vi "Valves2Linx.vi"(8 "error in (no error)":errorcluster, 11 "Valve (A1-C8),\n comma separated":string) -> (0 "error out":errorcluster, 2 "Array":bool[](array[boolean]), 3 "Array 2":i32[](array[numeric]))   [LabVIEW 2018]
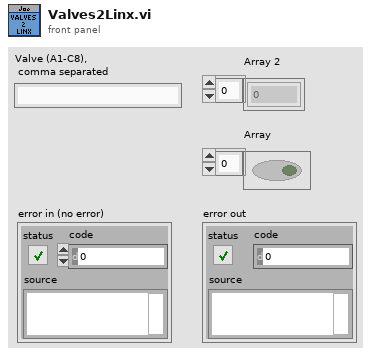
[diagram p1: front panel]
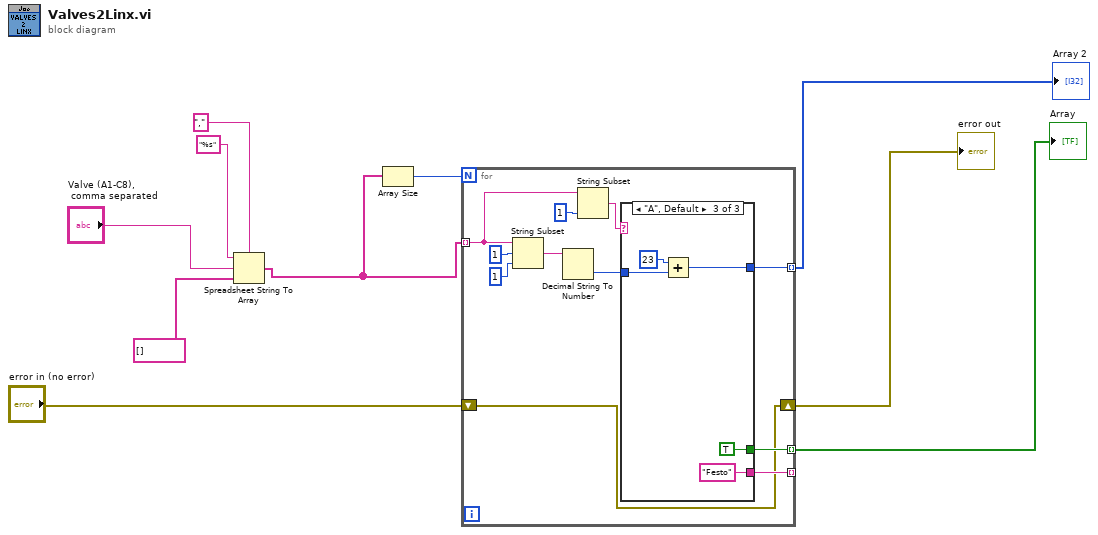
[diagram p0: block diagram]
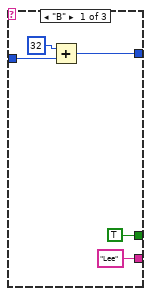
[diagram p2: hidden frame]
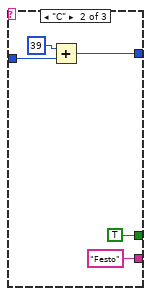
[diagram p3: hidden frame]
diagram:
  n1 = Spreadsheet String To Array(delimiter (Tab)=",", format string="%s", spreadsheet string="Valve (A1-C8),\n comma separated", array type (2D Dbl)=string[] []) -> (array=w2:string[])
  n2 = Array Size(array=w2) -> (size(s)=w6:i32)
  n3 = for {
    N: w6 -> [_]
    tunnel: w2 -> [w18] mode=indexing
    tunnel: [w13] -> w8 mode=indexing
    tunnel: [w14] -> _ mode=indexing
    tunnel: [w12] -> w7 mode=indexing
    shift-right: [w11] -> w10
    shift-left: "error in (no error)" -> [w11]
    n4 = String Subset(string=w18, offset (0)=1, length (rest)=1 ("length (rest)")) -> (substring=w16:string)
    n5 = Decimal String To Number(string=w16) -> (number=w15:i32)  [unwired: 2 in, 1 out]
    n6 = String Subset(string=w18, length (rest)=1 ("length (rest)")) -> (substring=w20:string)  [unwired: 1 in]
    n7 = case shown="\"A\", Default" w20 {
      tunnel: [w25 w30 w35] -> w12
      tunnel: w15 -> [w24 w29 w34]
      tunnel: ["Lee" "Festo" "Festo"] -> w14
      tunnel: [TRUE TRUE TRUE] -> w13
      frame "B" {
        n8 = Add(x=32, y=w24) -> (x+y=w25:i32)
      }
      frame "C" {
        n9 = Add(x=39, y=w29) -> (x+y=w30:i32)
      }
      frame "A", Default {
        n10 = Add(x=23, y=w34) -> (x+y=w35:i32)
      }
    }
  }
  "error out" <- w10
  "Array" <- w8
  "Array 2" <- w7
